vi "ClusterWithDotNetRef.vi"(10 "Cluster":T1={"Numeric"=0.0, "String"="", "Cluster"={"Numeric"=0.0, "Cluster"={"Boolean"=FALSE, "Ring"=11}}} {"Cluster"."Cluster"."Ring" items=["aaaa"=11, "bbbb"=22, "cccc"=33]}, 11 ".NET Refnum":refnum<k24>) -> (0 "error out":errorcluster, 3 "Has Expected Values":bool)   [LabVIEW 2013]
uses:
  NationalInstruments.TestStand.Interop.API
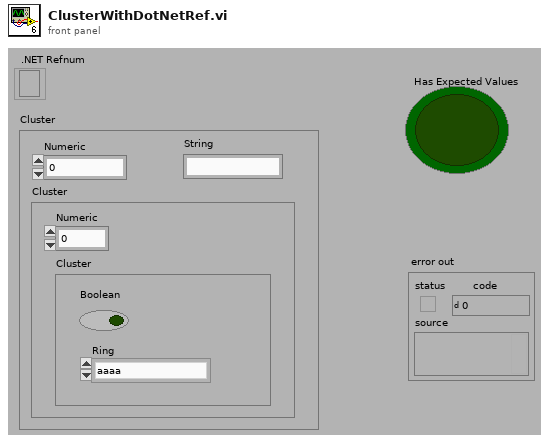
[diagram p1: front panel]
types:
  T1 = cluster{"Numeric":dbl, "String":string, "Cluster":cluster{"Numeric":dbl, "Cluster":cluster{"Boolean":bool, "Ring":u16}}}
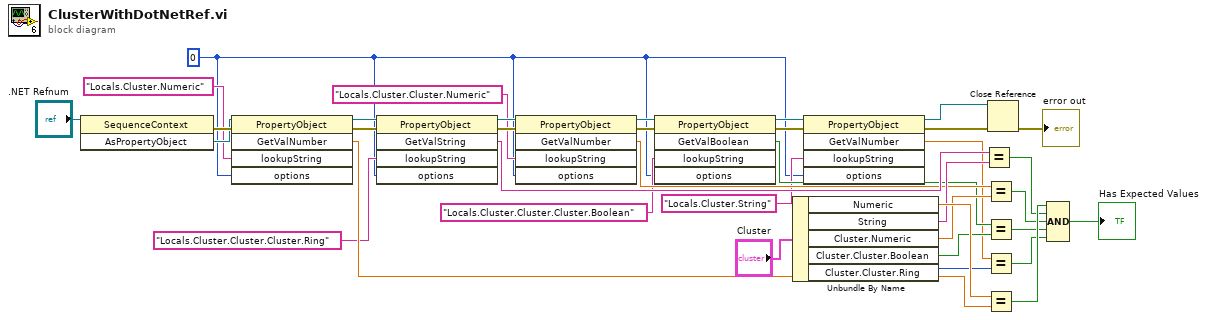
[diagram p0: block diagram]
diagram:
  w4 = 0 ("options")
  n1 = invoke class="SequenceContext" method="AsPropertyObject"(reference=".NET Refnum") -> (error out=w24:errorcluster, "AsPropertyObject"=w23:refnum<k24>)  [unwired: 2 in, 1 out]
  n2 = invoke class="PropertyObject" method="GetValNumber"(reference=w23, error in=w24, "lookupString"="Locals.Cluster.Numeric" ("Lookup String"), "options"=w4) -> (reference out=w18:refnum<k24>, error out=w19:errorcluster, "GetValNumber"=w21:dbl)  [unwired: 1 in, 2 out]
  n3 = invoke class="PropertyObject" method="GetValString"(reference=w18, error in=w19, "lookupString"="Locals.Cluster.Cluster.Cluster.Ring" ("Lookup String"), "options"=w4) -> (reference out=w16:refnum<k24>, error out=w15:errorcluster, "GetValString"=w17:string)  [unwired: 1 in, 2 out]
  n4 = invoke class="PropertyObject" method="GetValNumber"(reference=w16, error in=w15, "lookupString"="Locals.Cluster.Cluster.Numeric" ("Lookup String"), "options"=w4) -> (reference out=w12:refnum<k24>, error out=w11:errorcluster, "GetValNumber"=w13:dbl)  [unwired: 1 in, 2 out]
  n5 = invoke class="PropertyObject" method="GetValBoolean"(reference=w12, error in=w11, "lookupString"="Locals.Cluster.Cluster.Cluster.Boolean" ("Lookup String"), "options"=w4) -> (reference out=w8:refnum<k24>, error out=w7:errorcluster, "GetValBoolean"=w9:bool)  [unwired: 1 in, 2 out]
  n6 = Unbundle By Name("Cluster") -> ("Numeric"=w35:dbl, "String"=w33:string, "Cluster.Numeric"=w31:dbl, "Cluster.Cluster.Boolean"=w30:bool, "Cluster.Cluster.Ring"=w27:u16)
  n7 = invoke class="PropertyObject" method="GetValNumber"(reference=w8, error in=w7, "lookupString"="Locals.Cluster.String" ("Lookup String"), "options"=w4) -> (reference out=w2:refnum<k24>, error out=w3:errorcluster, "GetValNumber"=w5:dbl)  [unwired: 1 in, 2 out]
  n8 = Equal?(x=w17, y=w33) -> (x = y?=w32:bool)
  n9 = Equal?(x=w13, y=w31) -> (x = y?=w29:bool)
  n10 = Equal?(x=w9, y=w30) -> (x = y?=w28:bool)
  n11 = Equal?(x=w5, y=w27) -> (x = y?=w26:bool)
  n12 = Equal?(x=w35, y=w21) -> (x = y?=w34:bool)
  n13 = Close Reference(reference=w2, error in (no error)=w3) -> (error out=→"error out":errorcluster)
  n14 = Compound Arithmetic op=AND(w34, w32, w29, w28, w26) -> (→"Has Expected Values":bool)
